vi "gfitsio-hdu-dialog.vi"(7 "prompt (\"Select an HDU\")":string="Select an HDU", 8 "error in (no error)":errorcluster, 9 "select mode (new or existing)":enum32{"existing hdu", "new or existing hdu"}(ring)=enum."new or existing hdu", 10 "hdu type (ANY_HDU)":T1=-1 items=["ANY_HDU"=-1, "IMAGE_HDU"=0, "ASCII_TBL"=1, "BINARY_TBL"=2], 11 "gfits refnum":T2) -> (0 "error out":errorcluster, 1 "hdu number (0 if cancelled)":i32, 2 "hdu name (\"\" if cancelled)":string, 3 "dup gfits refnum":T2, 4 "cancelled":bool, 6 "exists":bool)   [LabVIEW 2019, in "gfitsio.lvlib"]
doc: "Displays a dialog box with which you can specify an HDU. You can use this dialog box to select existing HDUs or specify the name of a new HDU."
uses:
  gfitsio.lvlib
  gfitsio-refnum.ctl
  cfitsio-hdutypes.ctl
panel:
  out "Header":string
  in  "Existing HDUs List":i32(listbox) caption="Existing HDUs"
  in  "hdu name control":string caption="New HDU Name"
  in  "cancel":bool
  in  "ok":bool
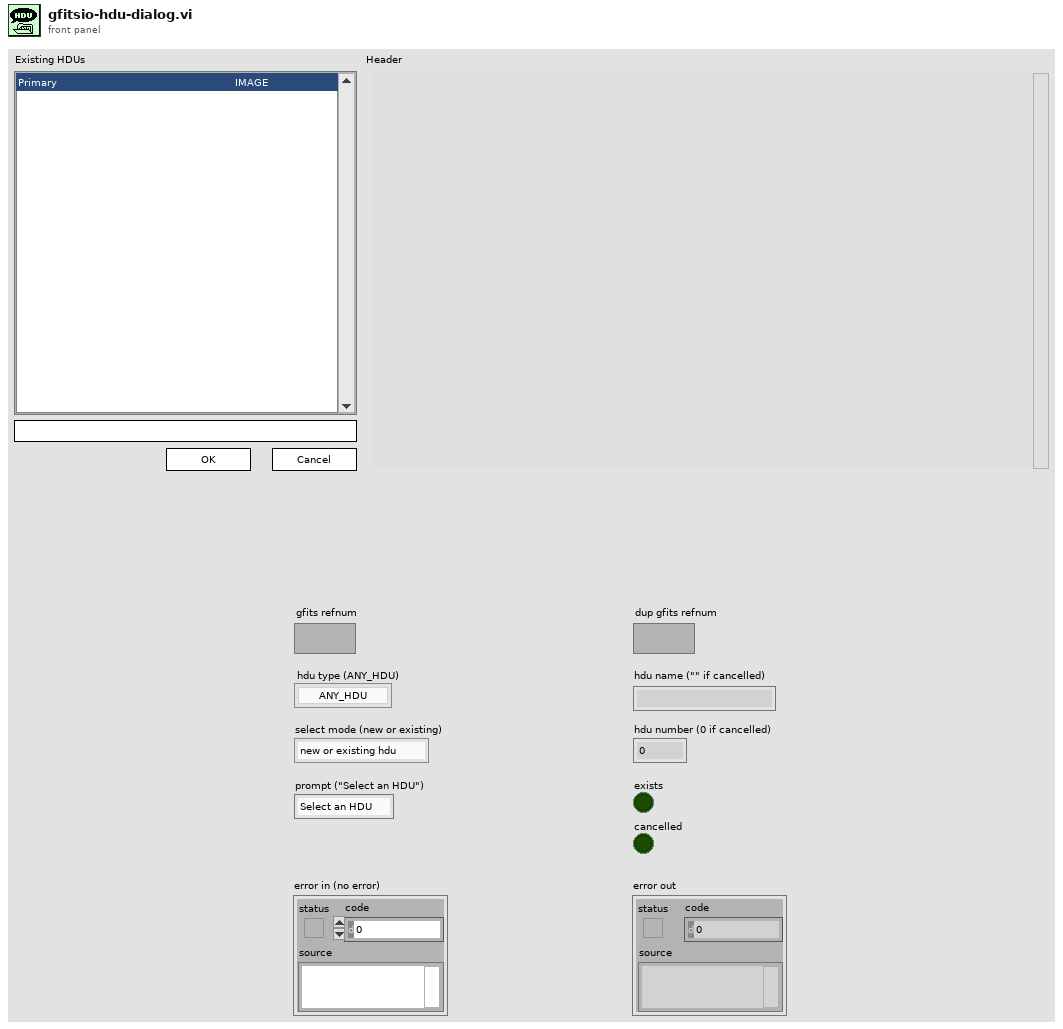
[diagram p1: front panel]
types:
  T1 = typedef "gfitsio.lvlib/cfitsio-hdutypes.ctl" = i32
  T2 = typedef "gfitsio.lvlib/gfitsio-refnum.ctl" = refnum<k1>
  T3 = typedef "LVRectTypeDef.ctl" = cluster{"Left":i16, "Top":i16, "Right":i16, "Bottom":i16}
  T4 = typedef "LVRowAndColumnUnsignedTypeDef.ctl" = cluster{"Row":u32, "Column":u32}
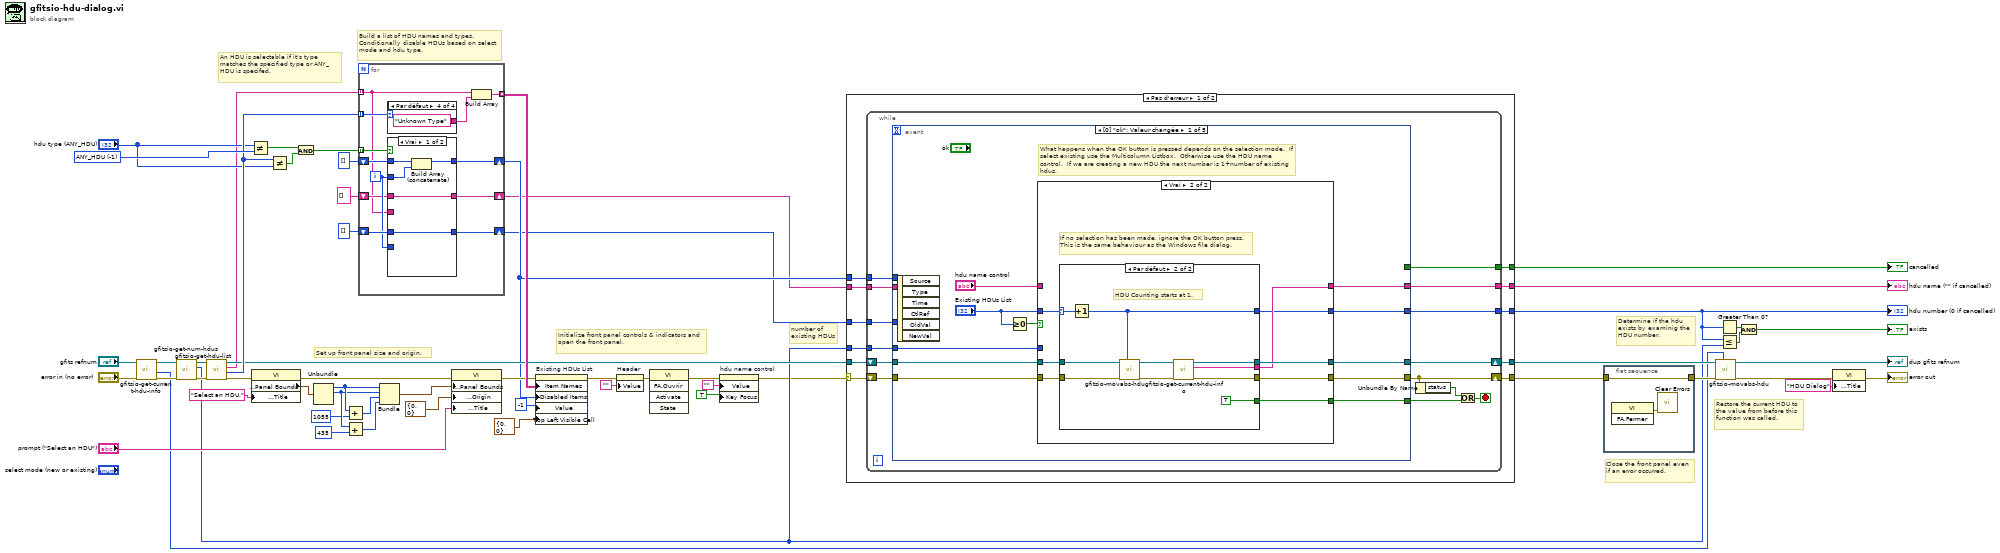
[diagram p0: block diagram]
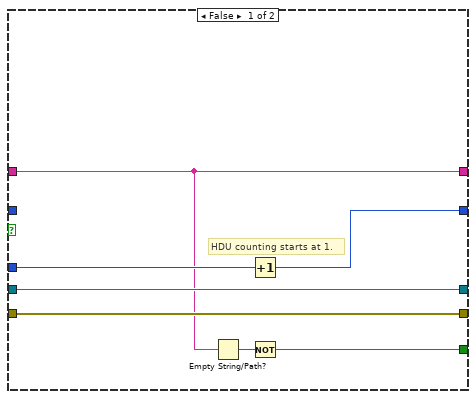
[diagram p2: hidden frame]
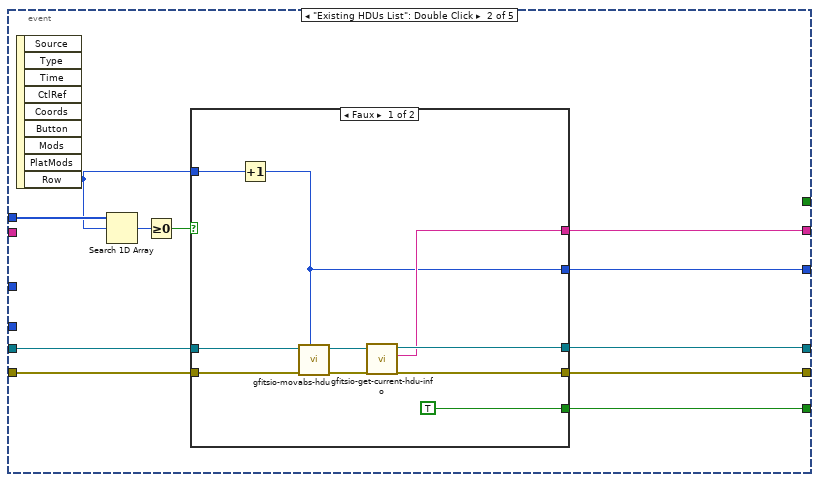
[diagram p4: hidden frame]
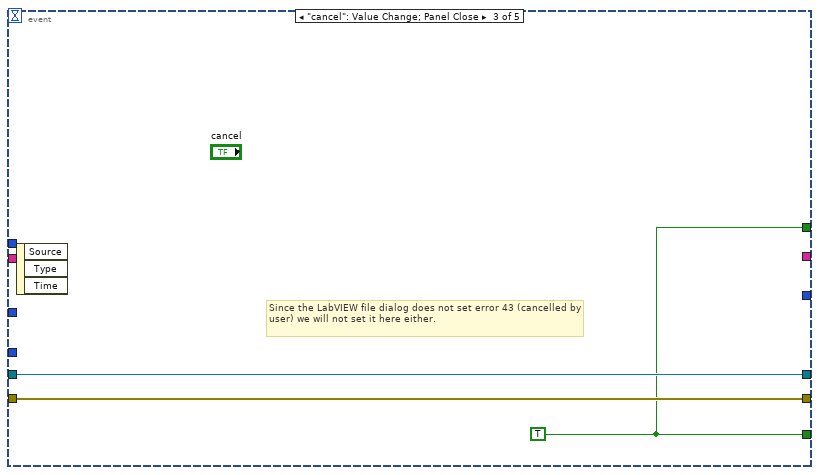
[diagram p6: hidden frame]
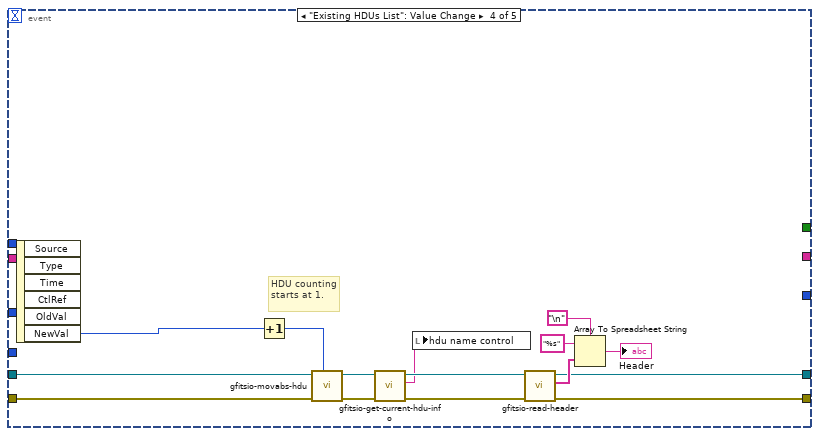
[diagram p7: hidden frame]
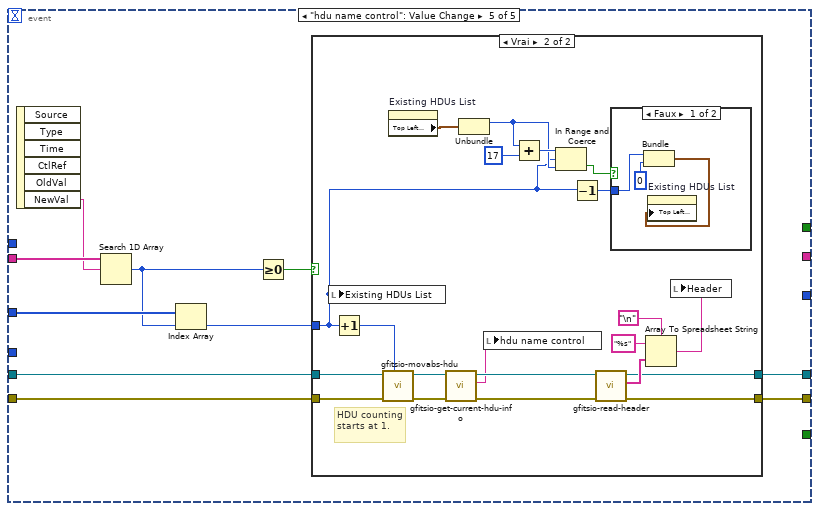
[diagram p8: hidden frame]
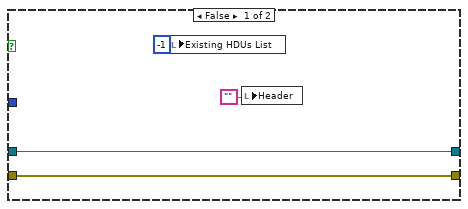
[diagram p9: hidden frame]
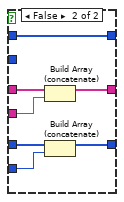
[diagram p12: hidden frame]
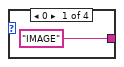
[diagram p13: hidden frame]
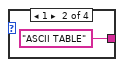
[diagram p14: hidden frame]
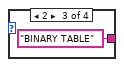
[diagram p15: hidden frame]
diagram:
  w54 = T1 -1 items=["ANY_HDU"=-1, "IMAGE_HDU"=0, "ASCII_TBL"=1, "BINARY_TBL"=2] ("hdu type")
  # "Determine if the hdu exists by examinig the HDU number."
  # "number of existing HDUs"
  # "An HDU is selectable if it's type matches the specified type or ANY_HDU is specifed."
  # "Initialize front panel controls & indicators and open the front panel."
  # "Set up front panel size and origin."
  # "Build a list of HDU names and types.  Conditionally disable HDUs based on select mode and hdu type."
  # "Restore the current HDU to the value from before this function was called."
  # "Close the front panel even if an error occurred."
  n1 = call "gfitsio-get-current-hdu-info.vi"("error in (no error)"="error in (no error)", "gfits refnum"="gfits refnum") -> ("error out"=w38:errorcluster, "hdu number"=w5:i32, "dup gfits refnum"=w37:T2)  [unwired: 5 in, 2 out]
  n2 = call "gfitsio-get-num-hdus.vi"("error in (no error)"=w38, "gfits refnum"=w37) -> ("error out"=w35:errorcluster, "number of hdus"=w16:i32, "dup gfits refnum"=w36:T2)  [unwired: 7 in]
  n3 = call "gfitsio-get-hdu-list.vi"("error in (no error)"=w35, "gfits refnum"=w36) -> ("error out"=w29:errorcluster, "hdu types"=w53:T1[], "hdu names"=w9:string[], "dup gfits refnum"=w34:T2)  [unwired: 6 in]
  n4 = Not Equal?(x="hdu type (ANY_HDU)", y=w54) -> (x != y?=w47:bool)
  n5 = property class="VI"(error in=w29, "Front Panel Window:Title"="Select an HDU.") -> (error out=w28:errorcluster, "Front Panel Window:Panel Bounds"=w46:T3)  [unwired: 1 in, 1 out]
  n6 = Not Equal?(x=w53, y="hdu type (ANY_HDU)") -> (x != y?=w48:bool[])
  n7 = And(x=w47, y=w48) -> (x .and. y?=w12:bool[])
  n8 = Unbundle(w46) -> ("Left"=w45:i16, "Top"=w44:i16)  [unwired: 2 out]
  n9 = Add(x=w45, y=i16 1055) -> (x+y=w41:i16)
  n10 = Add(x=w44, y=i16 435) -> (x+y=w42:i16)
  n11 = for {
    tunnel: w9 -> [w60] mode=indexing
    tunnel: w53 -> [w70] mode=indexing
    tunnel: [w71] -> w58 mode=indexing
    shift-right: [w66] -> w13
    shift-left: i32[] [] ("Disabled Items") -> [w67]
    tunnel: w12 -> [w68] mode=indexing
    shift-right: [w65] -> w7
    shift-left: i32[] [] ("Disabled Items") -> [w64]
    shift-right: [w61] -> w8
    shift-left: string[] [] ("Disabled Items") -> [w62]
    i -> [w63]
    n12 = case shown="Par défaut" w70 {
      tunnel: ["IMAGE" "ASCII TABLE" "BINARY TABLE" "Unknown Type"] -> w69
      frame 0 {
      }
      frame 1 {
      }
      frame 2 {
      }
      frame Default {
      }
    }
    n13 = case shown="Vrai" w68 {
      tunnel: w67 -> [w76 w77]
      tunnel: [w75 w77] -> w66
      tunnel: w63 -> [w74 _]
      tunnel: w64 -> [w73 w81]
      tunnel: [w73 w82] -> w65
      tunnel: w63 -> [_ w83]
      tunnel: w62 -> [w72 w80]
      tunnel: [w72 w79] -> w61
      tunnel: w60 -> [_ w78]
      frame True {
        n14 = Build Array (concatenate)(w76, w74) -> (w75:i32[])
      }
      frame False {
        n15 = Build Array (concatenate)(w80, w78) -> (w79:string[])
        n16 = Build Array (concatenate)(w81, w83) -> (w82:i32[])
      }
    }
    n17 = Build Array(w60, w69) -> (w71:string[])
  }
  n18 = Bundle("Left"=w45, "Top"=w44, w41, w42) -> (w31:cluster{"Left":i16, "Top":i16, i16, i16})  [unwired: 1 in]
  n19 = property class="VI"(error in=w28, "Front Panel Window:Panel Bounds"=w31, "Front Panel Window:Origin"=cluster{"Horizontal":i16, "Vertical":i16} {"Horizontal"=0, "Vertical"=0}, "Front Panel Window:Title"="prompt (\"Select an HDU\")") -> (error out=w26:errorcluster)  [unwired: 1 in, 1 out]
  n20 = property on="Existing HDUs List" class="ListeMCol (strict)"(error in=w26, "Item Names"=w58, "Disabled Items"=w13, "Value"=-1, "Top Left Visible Cell"=cluster{"Row":u32, "Column":u32} {"Row"=0, "Column"=0}) -> (error out=w25:errorcluster)  [unwired: 1 in, 1 out]
  n21 = property on="Header" class="Ch"(error in=w25, "Value"="") -> (error out=w24:errorcluster)  [unwired: 1 in, 1 out]
  n22 = invoke class="VI" method="FA.Ouvrir"(error in=w24) -> (error out=w22:errorcluster)  [unwired: 4 in, 4 out]
  n23 = property on="hdu name control" class="Ch"(error in=w22, "Value"="", "Key Focus"=TRUE) -> (error out=w15:errorcluster)  [unwired: 1 in, 1 out]
  n24 = case shown="Pas d'erreur" w15 {
    selector: w15 -> [w95 w231]
    tunnel: [w98 w230] -> w49
    tunnel: w34 -> [w97 w230]
    tunnel: [w96 w231] -> w59
    tunnel: [w94 _] -> w57
    tunnel: [w93 _] -> w56
    tunnel: [w92 _] -> w20
    tunnel: w16 -> [w91 _]
    tunnel: w8 -> [w90 _]
    tunnel: w13 -> [w89 _]
    tunnel: w7 -> [w88 _]
    frame No Error {
      n25 = while {
        shift-right: [w110] -> w98
        shift-left: w97 -> [w111]
        shift-right: [w108] -> w96
        shift-left: w95 -> [w112]
        tunnel: [w105] -> w94
        tunnel: [w104] -> w93
        tunnel: [w103] -> w92
        tunnel: w91 -> [w102]
        tunnel: w90 -> [w101]
        tunnel: w89 -> [w100]
        tunnel: w88 -> [w99]
        stop <- w106 stop-if-true
        n26 = event shown="[0] \"ok\": Valeur changée" {
          selector: _ -> [_ _ _ _ _]
          dyn-events: _ -> [_ _ _ _ _]
          timeout: _ -> [_ _ _ _ _]
          tunnel: w112 -> [w120 w160 w175 w190 w198]
          tunnel: [w117 w158 w175 w186 w196] -> w108
          tunnel: w111 -> [w119 w161 w176 w191 w199]
          tunnel: [w118 w159 w176 w187 w197] -> w110
          tunnel: [w121 w156 w174 _ _] -> w109
          tunnel: [w123 w157 _ _ _] -> w105
          tunnel: [_ _ w174 _ _] -> w104
          tunnel: [w122 w155 _ _ _] -> w103
          tunnel: w102 -> [w116 _ _ _ _]
          tunnel: w101 -> [_ _ _ _ w201]
          tunnel: w100 -> [_ w154 _ _ _]
          tunnel: w99 -> [_ _ _ _ w195]
          event "ok": Value Change {
            # "What happens when the OK button is pressed depends on the selection mode.  If select existing use the Multicolumn Listbox.  Otherwise use the HDU name control.  If we are creating a new HDU the next number is 1+number of existing hdus."
            n27 = event-data() -> ()  [unwired: 1 in, 6 out]
            n28 = Greater Or Equal To 0?(x="Existing HDUs List") -> (x >= 0?=w113:bool)
            n29 = case shown="Vrai" w113 {
              tunnel: [w126 w132] -> w123
              tunnel: [w127 w131] -> w122
              tunnel: [w124 w138] -> w121
              tunnel: w120 -> [w129 w134]
              tunnel: w119 -> [w130 w135]
              tunnel: [w130 w137] -> w118
              tunnel: [w129 w136] -> w117
              tunnel: "Existing HDUs List" -> [_ w133]
              tunnel: w116 -> [w128 _]
              tunnel: "hdu name control" -> [w126 _]
              frame False {
                # "HDU counting starts at 1."
                n30 = Empty String/Path?(string/path=w126) -> (empty?=w125:bool)
                n31 = Increment(x=w128) -> (x+1=w127:i32)
                n32 = Not(x=w125) -> (.not. x?=w124:bool)
              }
              frame True {
                # "If no selection has been made, ignore the OK button press.  This is the same behaviour as the Windows file dialog."
                n33 = case shown="Par défaut" w133 {
                  selector: w133 -> [_ w142]
                  tunnel: [_ TRUE] -> w138
                  tunnel: [w140 w150] -> w137
                  tunnel: [w139 w149] -> w136
                  tunnel: w135 -> [w140 w148]
                  tunnel: w134 -> [w139 w147]
                  tunnel: [_ w143] -> w132
                  tunnel: [_ w141] -> w131
                  frame -1 {
                  }
                  frame Default {
                    # "HDU Counting starts at 1."
                    n34 = Increment(x=w142) -> (x+1=w141:i32)
                    n35 = call "gfitsio-movabs-hdu.vi"("hdunum"=w141, "error in (no error)"=w147, "gfits refnum"=w148) -> ("error out"=w146:errorcluster, "dup gfits refnum"=w145:T2)  [unwired: 6 in, 1 out]
                    n36 = call "gfitsio-get-current-hdu-info.vi"("error in (no error)"=w146, "gfits refnum"=w145) -> ("error out"=w149:errorcluster, "hdu name"=w143:string, "dup gfits refnum"=w150:T2)  [unwired: 5 in, 2 out]
                  }
                }
              }
            }
          }
          event "Existing HDUs List": Double Click {
            n37 = event-data() -> ("Row"=w153:i32)  [unwired: 1 in, 8 out]
            n38 = Search 1D Array(1D array=w154, element=w153) -> (index of element=w152:i32)  [unwired: 1 in]
            n39 = Greater Or Equal To 0?(x=w152) -> (x >= 0?=w151:bool)
            n40 = case shown="Faux" w151 {
              tunnel: w161 -> [w171 w173]
              tunnel: w160 -> [w170 w172]
              tunnel: w153 -> [w169 _]
              tunnel: [w168 w173] -> w159
              tunnel: [w167 w172] -> w158
              tunnel: [w166 _] -> w157
              tunnel: [TRUE _] -> w156
              tunnel: [w162 _] -> w155
              frame False {
                n41 = Increment(x=w169) -> (x+1=w162:i32)
                n42 = call "gfitsio-movabs-hdu.vi"("hdunum"=w162, "error in (no error)"=w170, "gfits refnum"=w171) -> ("error out"=w164:errorcluster, "dup gfits refnum"=w163:T2)  [unwired: 6 in, 1 out]
                n43 = call "gfitsio-get-current-hdu-info.vi"("error in (no error)"=w164, "gfits refnum"=w163) -> ("error out"=w167:errorcluster, "hdu name"=w166:string, "dup gfits refnum"=w168:T2)  [unwired: 5 in, 2 out]
              }
              frame True {
              }
            }
          }
          event "cancel": Value Change; Panel Close {
            w174 = TRUE
            # "Since the LabVIEW file dialog does not set error 43 (cancelled by user) we will not set it here either."
            n44 = event-data() -> ()  [unwired: 1 in, 3 out]
          }
          event "Existing HDUs List": Value Change {
            # "HDU counting starts at 1."
            n45 = event-data() -> ("NewVal"=w189:i32)  [unwired: 1 in, 5 out]
            n46 = Increment(x=w189) -> (x+1=w177:i32)
            n47 = call "gfitsio-movabs-hdu.vi"("hdunum"=w177, "error in (no error)"=w190, "gfits refnum"=w191) -> ("error out"=w181:errorcluster, "dup gfits refnum"=w182:T2)  [unwired: 6 in, 1 out]
            n48 = call "gfitsio-get-current-hdu-info.vi"("error in (no error)"=w181, "gfits refnum"=w182) -> ("error out"=w180:errorcluster, "hdu name"=w178:string, "dup gfits refnum"=w179:T2)  [unwired: 5 in, 2 out]
            n49 = local write "hdu name control"(w178) -> ()
            n50 = call "gfitsio-read-header.vi"("error in (no error)"=w180, "gfits refnum"=w179) -> ("error out"=w186:errorcluster, "header"=w188:string[], "dup gfits refnum"=w187:T2)  [unwired: 7 in]
            n51 = Array To Spreadsheet String(delimiter (Tab)="\n", array=w188, 3:"%s" ("format string")) -> (spreadsheet string=→"Header":string)
          }
          event "hdu name control": Value Change {
            n52 = event-data() -> ("NewVal"=w200:string)  [unwired: 1 in, 5 out]
            n53 = Search 1D Array(1D array=w201, element=w200) -> (index of element=w194:i32)  [unwired: 1 in]
            n54 = Index Array(array=w195, index=w194) -> (element=w192:i32)
            n55 = Greater Or Equal To 0?(x=w194) -> (x >= 0?=w193:bool)
            n56 = case shown="Vrai" w193 {
              tunnel: w199 -> [w205 w218]
              tunnel: w198 -> [w204 w217]
              tunnel: [w205 w216] -> w197
              tunnel: [w204 w215] -> w196
              tunnel: w192 -> [_ w209]
              frame False {
                n57 = local write "Existing HDUs List"(-1 ("Existing HDUs List")) -> ()
                n58 = local write "Header"("") -> ()
              }
              frame True {
                # "HDU counting starts at 1."
                n59 = local write "Existing HDUs List"(w209) -> ()
                n60 = Increment(x=w209) -> (x+1=w206:i32)
                n61 = call "gfitsio-movabs-hdu.vi"("hdunum"=w206, "error in (no error)"=w217, "gfits refnum"=w218) -> ("error out"=w222:errorcluster, "dup gfits refnum"=w223:T2)  [unwired: 6 in, 1 out]
                n62 = property on="Existing HDUs List" class="ListeMCol (strict)"() -> ("Top Left Visible Cell"=w213:T4)  [unwired: 2 in, 2 out]
                n63 = call "gfitsio-get-current-hdu-info.vi"("error in (no error)"=w222, "gfits refnum"=w223) -> ("error out"=w221:errorcluster, "hdu name"=w219:string, "dup gfits refnum"=w220:T2)  [unwired: 5 in, 2 out]
                n64 = Unbundle(w213) -> ("Row"=w210:u32)  [unwired: 1 out]
                n65 = local write "hdu name control"(w219) -> ()
                n66 = Add(x=w210, y=u32 17) -> (x+y=w211:u32)
                n67 = In Range and Coerce(upper limit=w211, x=w209, lower limit=w210) -> (In Range?=w208:bool)  [unwired: 1 out]
                n68 = Decrement(x=w209) -> (x-1=w207:i32)
                n69 = call "gfitsio-read-header.vi"("error in (no error)"=w221, "gfits refnum"=w220) -> ("error out"=w215:errorcluster, "header"=w226:string[], "dup gfits refnum"=w216:T2)  [unwired: 7 in]
                n70 = case shown="Faux" w208 {
                  tunnel: w207 -> [w229 _]
                  frame False {
                    n71 = Bundle(w229, 0) -> (w227:cluster{i32, i32})  [unwired: 1 in]
                    n72 = property on="Existing HDUs List" class="ListeMCol (strict)"("Top Left Visible Cell"=w227) -> ()  [unwired: 2 in, 2 out]
                  }
                  frame True {
                  }
                }
                n73 = Array To Spreadsheet String(delimiter (Tab)="\n", array=w226, 3:"%s" ("format string")) -> (spreadsheet string=w214:string)
                n74 = local write "Header"(w214) -> ()
              }
            }
          }
        }
        n75 = Unbundle By Name(w108) -> ("status"=w107:bool)
        n76 = Or(x=w107, y=w109) -> (x .or. y?=w106:bool)
      }
    }
    frame Error {
    }
  }
  "hdu name (\"\" if cancelled)" <- w57
  "cancelled" <- w56
  "hdu number (0 if cancelled)" <- w20
  n77 = flat-sequence {
    tunnel: [w233] -> w51
    tunnel: w59 -> [w233]
    frame #0 {
      n78 = invoke class="VI" method="FA.Fermer"() -> (error out=w232:errorcluster)  [unwired: 3 in, 2 out]
      n79 = call <vilib>:"Clear Errors.vi"("error in (no error)"=w232) -> ()  [unwired: 5 in, 2 out]
    }
  }
  n80 = call "gfitsio-movabs-hdu.vi"("hdunum"=w5, "error in (no error)"=w51, "gfits refnum"=w49) -> ("error out"=w3:errorcluster, "dup gfits refnum"=→"dup gfits refnum":T2)  [unwired: 6 in, 1 out]
  n81 = Greater Than 0?(x=w20) -> (x > 0?=w19:bool)
  n82 = Less Or Equal?(x=w20, y=w16) -> (x <= y?=w18:bool)
  n83 = And(x=w19, y=w18) -> (x .and. y?=→"exists":bool)
  n84 = property class="VI"(error in=w3, "Front Panel Window:Title"="HDU Dialog") -> (error out=→"error out":errorcluster)  [unwired: 1 in, 1 out]
